vi "题目一.vi"() -> ()   [LabVIEW 2017]
panel:
  out "7（X0=10,dx=2,Y）多条曲线":cluster{i32, i32, cluster{dbl[]}[]}(graph)
  out "6（X0=10,dx=2,Y）多条曲线":cluster{i32, i32, dbl[][]}(graph)
  out "5（X0=10,dx=2,Y）多条曲线":cluster{i32, i32, dbl[]}[](graph)
  out "4（X0=10,dx=2,Y）单条曲线":cluster{i32, i32, dbl[]}(graph)
  out "3（Y）多条曲线":cluster{dbl[]}[](graph)
  out "2（Y）多条曲线":dbl[][](graph)
  out "1（Y）单条曲线":dbl[](graph)
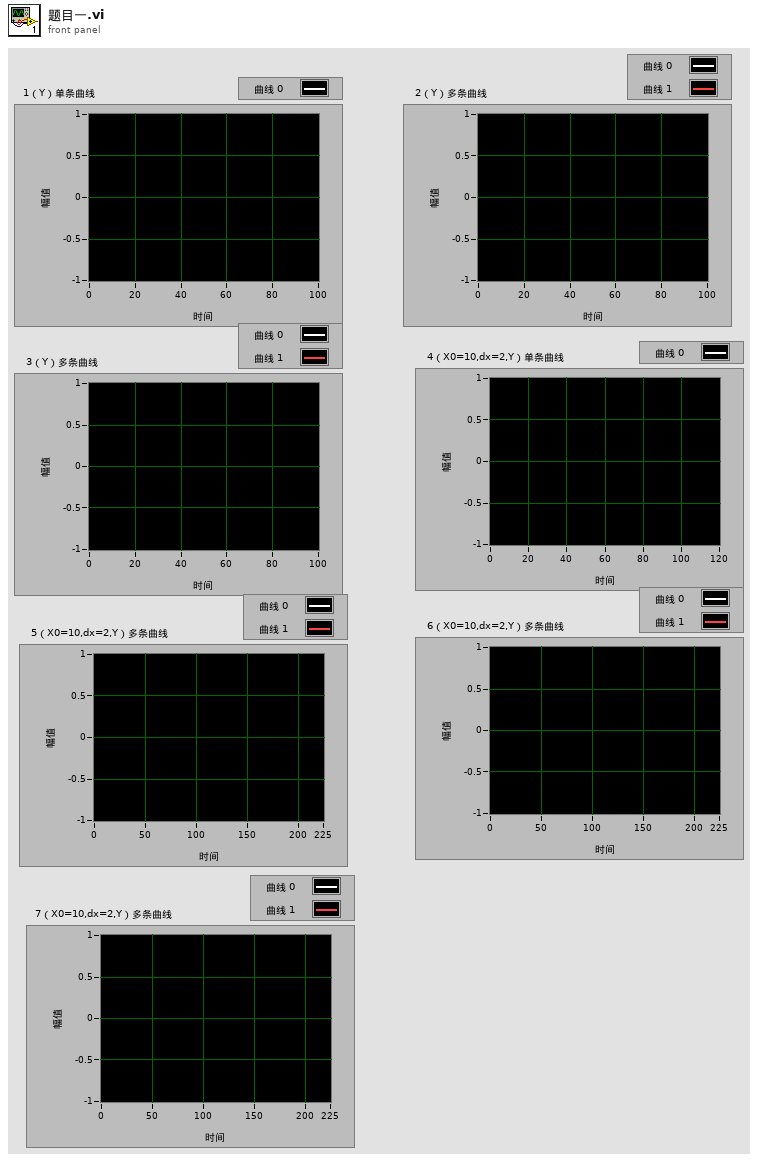
[diagram p1: front panel]
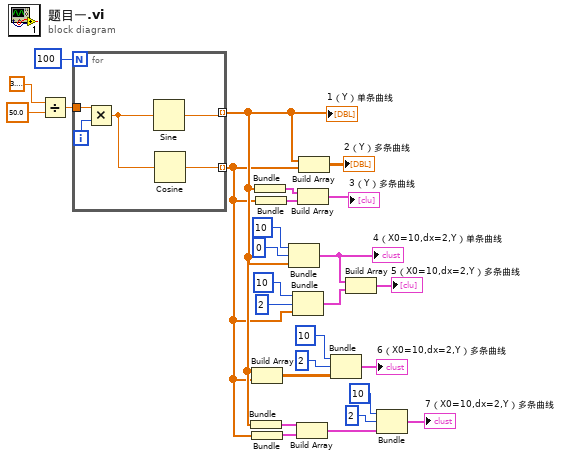
[diagram p0: block diagram]
diagram:
  n1 = Divide(x=3.141592653589793, y=50.0) -> (x/y=w24:dbl)
  n2 = for {
    N: 100 -> [_]
    tunnel: w24 -> [w32]
    tunnel: [w29] -> w8 mode=indexing
    tunnel: [w28] -> w7 mode=indexing
    i -> [w31]
    n3 = Multiply(x=w32, y=w31) -> (x*y=w30:dbl)
    n4 = Sine(x=w30) -> (sin(x)=w29:dbl)
    n5 = Cosine(x=w30) -> (cos(x)=w28:dbl)
  }
  "1（Y）单条曲线" <- w8
  n6 = Bundle(w8) -> (w6:cluster{dbl[]})  [unwired: 1 in]
  n7 = Build Array(w8, w7) -> (w12:dbl[][])
  n8 = Bundle(w7) -> (w5:cluster{dbl[]})  [unwired: 1 in]
  n9 = Bundle(w8) -> (w23:cluster{dbl[]})  [unwired: 1 in]
  n10 = Bundle(w7) -> (w22:cluster{dbl[]})  [unwired: 1 in]
  n11 = Bundle(10, 0, w8) -> (w14:cluster{i32, i32, dbl[]})  [unwired: 1 in]
  "4（X0=10,dx=2,Y）单条曲线" <- w14
  n12 = Bundle(10, 2, w7) -> (w15:cluster{i32, i32, dbl[]})  [unwired: 1 in]
  n13 = Build Array(w6, w5) -> (w4:cluster{dbl[]}[])
  n14 = Build Array(w23, w22) -> (→"3（Y）多条曲线":cluster{dbl[]}[])
  n15 = Build Array(w8, w7) -> (→"2（Y）多条曲线":dbl[][])
  n16 = Bundle(10, 2, w12) -> (→"6（X0=10,dx=2,Y）多条曲线":cluster{i32, i32, dbl[][]})  [unwired: 1 in]
  n17 = Build Array(w14, w15) -> (→"5（X0=10,dx=2,Y）多条曲线":cluster{i32, i32, dbl[]}[])
  n18 = Bundle(10, 2, w4) -> (→"7（X0=10,dx=2,Y）多条曲线":cluster{i32, i32, cluster{dbl[]}[]})  [unwired: 1 in]
